vi "Get SMO Database Paths.vi"(5 "getAll Cluster":variant, 7 "Paths":string="llab_038:d000(TEST_TABLE--Temperature(Kelvin))\nllab_038:d002(TEST_TABLE--voltage 2(volts))\nllab_038:b000(TEST_TABLE--ON?())\nllab_038:v001(TEST_TABLE--sample())", 8 "error in (no error)":errorcluster, 11 "Inst.RP100 in":refnum<class "Inst.RP100.lvclass">) -> (0 "error out":errorcluster, 2 "Paths":string, 3 "Inst.RP100 out":refnum<class "Inst.RP100.lvclass">)   [LabVIEW 2019, in "Inst.RP100.lvlib" / "Inst.RP100.lvclass"]
uses:
  Inst.RP100.lvclass
  Typedefs/Inst.RP100.getAll--Cluster.ctl
  <userlib>/LevyLab/LV-Data/LV-Data.PG/LV-Data.PGSQL.lvclass
  <userlib>/LevyLab/LV-Data/LV-Data.PG/API/Write Variable (one-row).vi
  <userlib>/LevyLab/Instrument Framework/Instrument Types/Strain/Instrument.Strain.lvclass
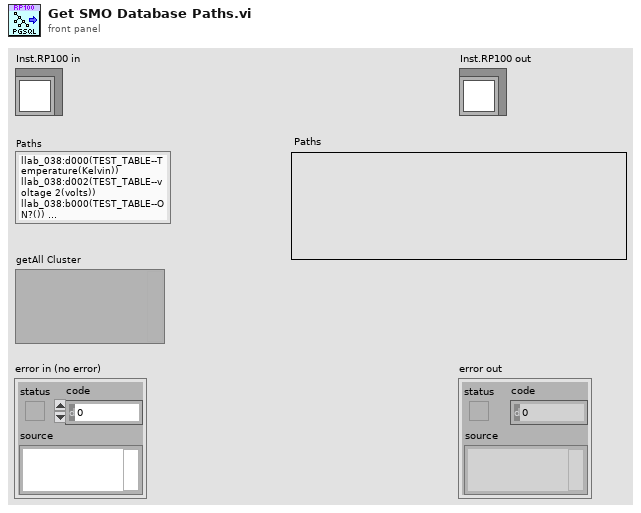
[diagram p1: front panel]
types:
  T1 = typedef "Inst.RP100.lvlib/Inst.RP100.lvclass/Inst.RP100.getAll--Cluster.ctl" = cluster{"OutputStateCh1":string, "OutputStateCh2":string, "LevelCh1":dbl, "LevelCh2":dbl, "SlewCh1":dbl, "SlewCh2":dbl, "MeasuredVCh1":dbl, "MeasuredVCh2":dbl, "MeasuredICh1":dbl, "MeasuredICh2":dbl}
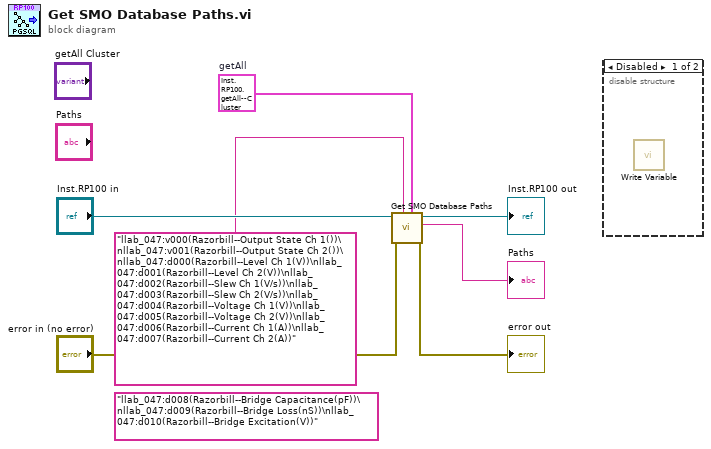
[diagram p0: block diagram]
diagram:
  (unwired) "llab_047:d008(Razorbill--Bridge Capacitance(pF))\nllab_047:d009(Razorbill--Bridge Loss(nS))\nllab_047:d010(Razorbill--Bridge Excitation(V))" ("Paths")
  w2 = T1 {"OutputStateCh1"="", "OutputStateCh2"="", "LevelCh1"=0.0, "LevelCh2"=0.0, "SlewCh1"=0.0, "SlewCh2"=0.0, "MeasuredVCh1"=0.0, "MeasuredVCh2"=0.0, "MeasuredICh1"=0.0, "MeasuredICh2"=0.0}  # getAll
  n1 = call-parent "Get SMO Database Paths.vi"("getAll Cluster"=w2, "Default Paths"="llab_047:v000(Razorbill--Output State Ch 1())\nllab_047:v001(Razorbill--Output State Ch 2())\nllab_047:d000(Razorbill--Level Ch 1(V))\nllab_047:d001(Razorbill--Level Ch 2(V))\nllab_047:d002(Razorbill--Slew Ch 1(V/s))\nllab_047:d003(Razorbill--Slew Ch 2(V/s))\nllab_047:d004(Razorbill--Voltage Ch 1(V))\nllab_047:d005(Razorbill--Voltage Ch 2(V))\nllab_047:d006(Razorbill--Current Ch 1(A))\nllab_047:d007(Razorbill--Current Ch 2(A))" ("Paths"), "error in (no error)"="error in (no error)", "Instrument in"="Inst.RP100 in") -> ("error out"=→"error out":errorcluster, "Paths"=→"Paths":string, "Instrument out"=→"Inst.RP100 out":refnum<class "Inst.RP100.lvclass">)  [unwired: 5 in]
  n2 = disable-structure shown="Disabled" {
    frame Disabled {
      n3 = call-poly <userlib>:"Write Variable.vi"() -> ()  [unwired: 8 in, 4 out]
    }
    frame Enabled {
    }
  }
